vi "ActionVIOnDeleteRequestMainPage.vi"(6 "Refs that are about to get deleted":T1[](array[typedef]) format="%.0x", 8 "error in (no error)":errorcluster, 11 "Item Ref in":T1 format="%.0x") -> (0 "error out":errorcluster, 1 "Discard reason":string, 2 "Additional items to delete":T1[](array[typedef]) format="%.0x", 3 "Item Ref out":T1 format="%.0x", 4 "Discard delete request?":bool)   [LabVIEW 2014]
uses:
  <vilib>/NI Veristand/Custom Device API/Custom Device Item Ref.ctl
  <vilib>/NI Veristand/Custom Device API/Custom Device API.lvlib
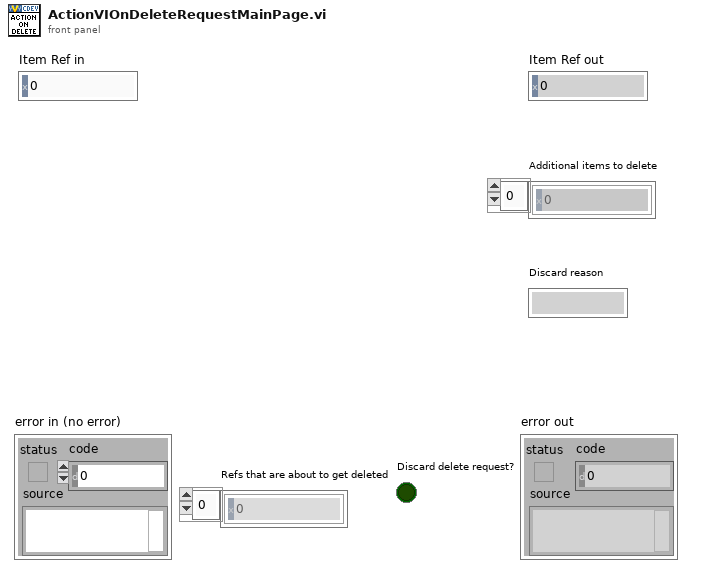
[diagram p1: front panel]
types:
  T1 = typedef "Custom Device API.lvlib/Custom Device Item Ref.ctl" = u64
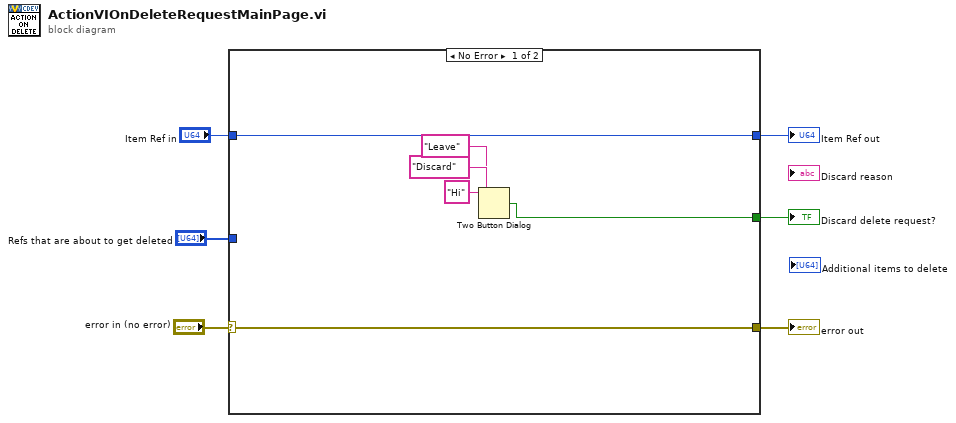
[diagram p0: block diagram]
diagram:
  n1 = case shown="No Error" "error in (no error)" {
    selector: "error in (no error)" -> [w12 w14]
    tunnel: [w12 w14] -> w5
    tunnel: "Item Ref in" -> [w11 w13]
    tunnel: [w11 w13] -> w3
    tunnel: "Refs that are about to get deleted" -> [_ _]
    tunnel: [w7 _] -> w1
    frame No Error {
      n2 = Two Button Dialog(message="Hi", 1:"Leave" ("F button name (\"Cancel\")"), 2:"Discard" ("T button name (\"OK\")")) -> (T button?=w7:bool)
    }
    frame Error {
    }
  }
  "error out" <- w5
  "Item Ref out" <- w3
  "Discard delete request?" <- w1
